vi "Delete Group.vi"(8 "error in":errorcluster, 9 "Selected Group":T1, 11 "Chassis Cfg":refnum<class "ChassisCfg.lvclass">) -> (0 "error out":errorcluster, 1 "Selected Group":T1, 2 "Deleted Grp":refnum<class "ChanGrp.lvclass">, 3 "Chassis Cfg":refnum<class "ChassisCfg.lvclass">)   [LabVIEW 2012, in "Configuration Grandmaster.lvlib" / "ChassisCfg.lvclass"]
uses:
  ChassisCfg.lvclass
  Common/Controls/Selected Group.ctl
  Common/Controls/TE_Designator.ctl
  Class Chan Group/ChanGrp.lvclass
  ChassisCfg.lvclass/ChassisCfg.ctl
  Class Timing Group/TimingGrp.lvclass
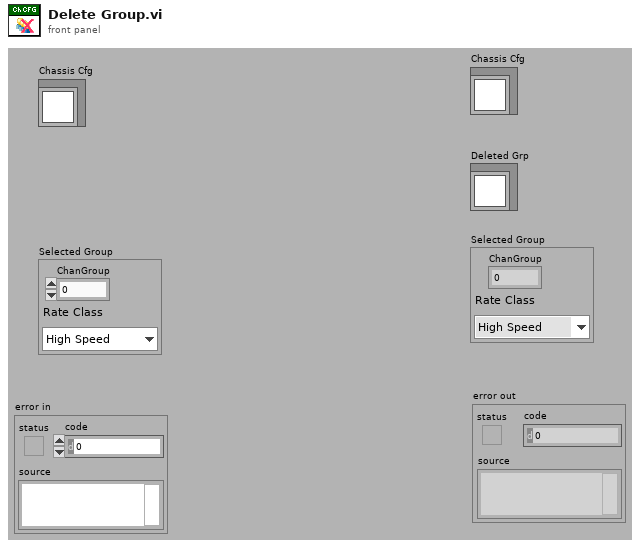
[diagram p1: front panel]
types:
  T1 = typedef "Selected Group.ctl" = cluster{"ChanGroup":i32, "Rate Class":T2}
  T2 = typedef "TE_Designator.ctl" = enum16{"High Speed", "Low Speed"}
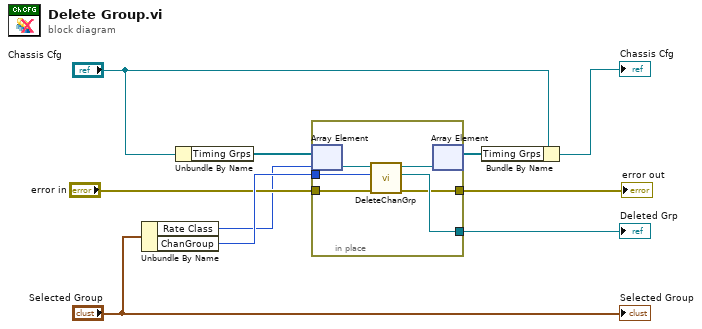
[diagram p0: block diagram]
diagram:
  n1 = Unbundle By Name("Selected Group") -> ("Rate Class"=w2:T2, "ChanGroup"=w8:i32)
  n2 = Unbundle By Name("Chassis Cfg") -> ("Timing Grps"=w3:refnum<class "TimingGrp.lvclass">[])
  n3 = in-place {
    in-place-border: w8 -> [w16]
    in-place-border: [w15] -> w6
    in-place-border: "error in" -> [w14]
    in-place-border: [w13] -> w4
    n4 = in-place-array #1(w3, w2) -> (w12:refnum<class "TimingGrp.lvclass">)
    n5 = call "DeleteChanGrp.vi"("error in"=w14, "ChanGroup"=w16, "TimingGrp in"=w12) -> ("error out"=w13:errorcluster, "ChanGrp.lvclass"=w15:refnum<class "ChanGrp.lvclass">, "TimingGrp in"=w11:refnum<class "TimingGrp.lvclass">)  [unwired: 6 in]
    n6 = in-place-array #1(w11) -> (w1:refnum<class "TimingGrp.lvclass">[])  [unwired: 1 out]
  }
  "Deleted Grp" <- w6
  "error out" <- w4
  n7 = Bundle By Name(cluster="Chassis Cfg", "Timing Grps"=w1) -> (→"Chassis Cfg":refnum<class "ChassisCfg.lvclass">)
  "Selected Group" <- "Selected Group"
